vi "checkFinishPenaltyEnemyPlayVSS.vi"(8 "error in (no error)":errorcluster, 9 "last command_interpreted":T1, 10 "Game in":refnum<class "Game.lvclass">, 11 "PenaltyEnemyPlayVSS in":refnum<class "PenaltyEnemyPlayVSS.lvclass">) -> (0 "error out":errorcluster, 2 "result":bool, 3 "PenaltyEnemyPlayVSS out":refnum<class "PenaltyEnemyPlayVSS.lvclass">)   [LabVIEW 2018, in "PenaltyEnemyPlayVSS.lvclass"]
uses:
  PenaltyEnemyPlayVSS.lvclass
  Referee_class/command_interpreted.ctl
  Game_class/Game.lvclass
  Game_class/Game.lvclass/Game.ctl
  Referee_class/Referee.lvclass/Referee.ctl
  Events_class/Events.lvclass/Events.ctl
  Game_class/Read Referee.vi
  Game_class/Read EventsRef.vi
  Events_class/Read ball_out.vi
  Events_class/Read touch.vi
  Events_class/Read id_touch.vi
  Referee_class/Read command_interpreted.vi
  Referee_class/Referee.lvclass
  Events_class/Events.lvclass
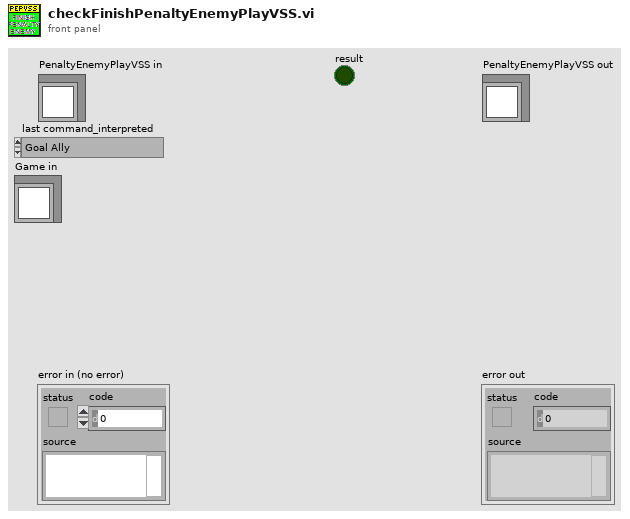
[diagram p1: front panel]
types:
  T1 = typedef "command_interpreted.ctl" = enum16{"Goal Ally", "Goal Enemy", "Ball Placement Enemy", "Ball Placement Ally", "Normal Half Time", "Extra Time  Break", "Extra Half Time", "None", "Post Game", "PKA Normal Start", "Prepare Kickoff Ally", "PKE Normal Start", "Prepare Kickoff Enemy", "Force Start", "Halt", "Timeout", "Prepare Penalty Ally", "Prepare Penalty Enemy", "PPA NormalStart", "PPE Normal Start", "Indirect Free Ally", "Direct Free Enemy", "Direct Free Ally", "Indirect Free Enemy", "Stop"}
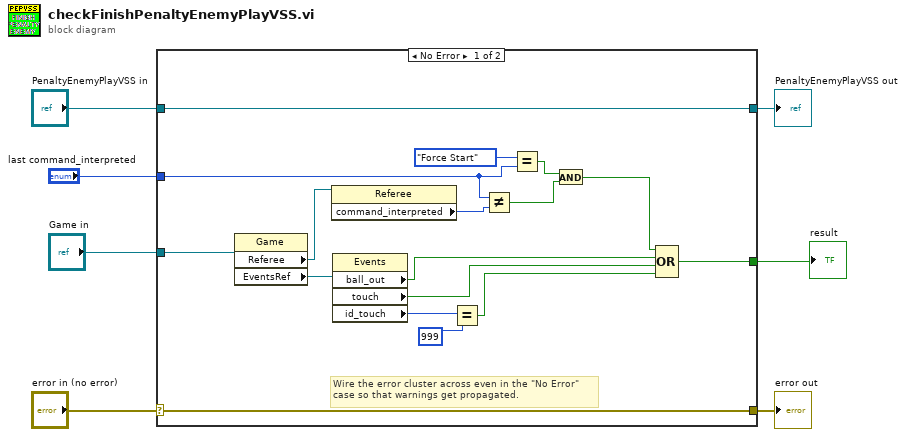
[diagram p0: block diagram]
diagram:
  n1 = case shown="No Error" "error in (no error)" {
    selector: "error in (no error)" -> [w23 w26]
    tunnel: [w23 w26] -> w6
    tunnel: [w24 w25] -> w4
    tunnel: "PenaltyEnemyPlayVSS in" -> [w24 w25]
    tunnel: "Game in" -> [w22 _]
    tunnel: "last command_interpreted" -> [w12 _]
    tunnel: [w8 _] -> w1
    frame No Error {
      # "Wire the error cluster across even in the \"No Error\"\ncase so that warnings get propagated."
      n2 = property class="Game"(reference=w22) -> ("Referee"=w15:refnum<class "Referee.lvclass">, "EventsRef"=w21:refnum<class "Events.lvclass">)  [unwired: 1 in, 2 out]
      n3 = property class="Referee"(reference=w15) -> ("command_interpreted"=w11:T1)  [unwired: 1 in, 2 out]
      n4 = property class="Events"(reference=w21) -> ("ball_out"=w16:bool, "touch"=w18:bool, "id_touch"=w20:i32)  [unwired: 1 in, 2 out]
      n5 = Equal?(x=w20, y=999) -> (x = y?=w17:bool)
      n6 = Not Equal?(x=w12, y=w11) -> (x != y?=w10:bool)
      n7 = Equal?(x=command_interpreted."Force Start" ("command_interpreted"), y=w12) -> (x = y?=w13:bool)
      n8 = And(x=w13, y=w10) -> (x .and. y?=w9:bool)
      n9 = Compound Arithmetic op=OR(w9, w16, w18, w17) -> (w8:bool)
    }
    frame Error {
    }
  }
  "error out" <- w6
  "PenaltyEnemyPlayVSS out" <- w4
  "result" <- w1
